vi "CAN BOOT Execute App.vi"(9 "NAD":u8, 10 "CANIndex":i32, 11 "DevHandle":i32) -> (3 "function return":i32)   [LabVIEW 2010, in "can_bootloader.lvlib"]
doc: "int WINAPI CAN_BOOT_ExecuteApp(int DevHandle,int CANIndex,unsigned char NAD);"
uses:
  can_bootloader.lvlib
  USB2XXX/trunk/USB2XXX/USB2XXX/vs2010/Release/USB2XXX.dll
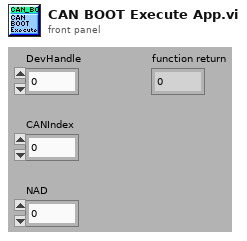
[diagram p1: front panel]
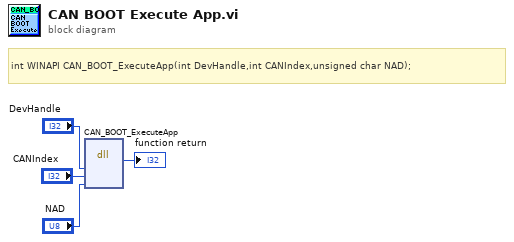
[diagram p0: block diagram]
diagram:
  # "int WINAPI CAN_BOOT_ExecuteApp(int DevHandle,int CANIndex,unsigned char NAD);"
  n1 = dll-call lib="E:/OtherWork/STM32/USB2XXX/trunk/USB2XXX/USB2XXX/vs2010/Release/USB2XXX.*" fn="CAN_BOOT_ExecuteApp"("DevHandle"="DevHandle", "CANIndex"="CANIndex", "NAD"="NAD") -> (→"function return":i32)  [unwired: 6 in, 2 out]
